vi "Map TS Name to Project TI Name.vi"(11 "target structure name":string) -> (3 "project targetitem name":string)   [LabVIEW 2020, in "NI_TargetHelper.lvlib"]
uses:
  <vilib>/TargetSupport/NI_TargetHelper/NI_TargetHelper.lvlib
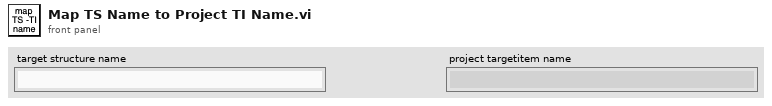
[diagram p1: front panel]
types:
  T1 = cluster{"name":string, "owner":bool, "none":bool, "one":bool, "auto":bool, "choose":bool, "opt#":bool, "ipaddr":bool, "[loc,]mod":bool, "TSname":string}[]
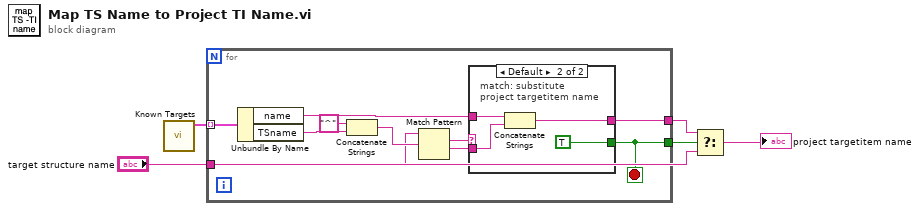
[diagram p0: block diagram]
diagram:
  n1 = call <vilib>:"Known Targets.vi"() -> ("targets        project targetItem name              menu to use                    fpga sub                                           suffix info"=w5:T1)  [unwired: 11 in]
  n2 = for {
    tunnel: w5 -> [w15] mode=indexing
    tunnel: "target structure name" -> [w12]
    tunnel: [w8] -> w4
    tunnel: [w7] -> w3
    stop <- w7 stop-if-true
    n3 = Unbundle By Name(w15) -> ("name"=w9:string, "TSname"=w6:string)
    n4 = Concatenate Strings("^" ("string"), w6) -> (w13:string)
    n5 = Match Pattern(string=w12, regular expression=w13) -> (match substring=w11:string, after substring=w10:string)  [unwired: 1 in, 2 out]
    n6 = case shown="Default" w11 {
      tunnel: w10 -> [_ w18]
      tunnel: w9 -> [_ w19]
      tunnel: [_ w17] -> w8
      tunnel: [_ TRUE] -> w7
      frame "" {
        # "no match"
      }
      frame Default {
        # "match: substitute\nproject targetitem name"
        n7 = Concatenate Strings(w19, w18) -> (w17:string)
      }
    }
  }
  n8 = Select(t=w4, s=w3, f="target structure name") -> (s? t:f=→"project targetitem name":string)
